vi "Handle Request.vi"(7 "Processing In":refnum<class "Processing.lvclass">, 11 "SSE Handler in":refnum<class "SSE Handler.lvclass">) -> (0 "error out":errorcluster, 5 "Processing":refnum<class "Processing.lvclass">)   [LabVIEW 2020, in "HTTP Server.lvlib" / "SSE Handler.lvclass"]
uses:
  SSE Handler.lvclass
  Processing/Processing.lvclass
  Processing/Processing.lvclass/Processing.ctl
  SSE Manager/SSE Manager.lvclass
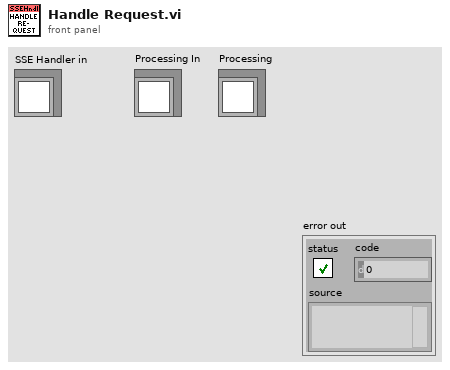
[diagram p1: front panel]
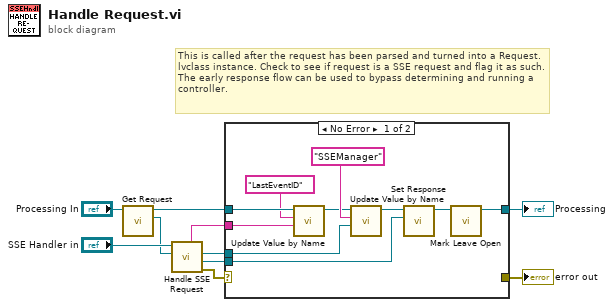
[diagram p0: block diagram]
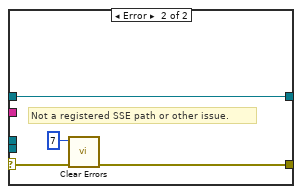
[diagram p2: hidden frame]
diagram:
  # "This is called after the request has been parsed and turned into a Request.lvclass instance. Check to see if request is a SSE request and flag it as such. The early response flow can be used to bypass determining and running a controller."
  n1 = call "Get Request.vi"("Processing in"="Processing In") -> ("Request"=w6:refnum<class "Request.lvclass">, "Processing out"=w9:refnum<class "Processing.lvclass">)  [unwired: 9 in]
  n2 = call "Handle SSE Request.vi"("Request"=w6, "SSE Handler in"="SSE Handler in") -> ("error out"=w5:errorcluster, "Response"=w4:refnum<class "Response.lvclass">, "SSE Manager"=w3:refnum<class "SSE Manager.lvclass">, "Last Event ID"=w2:string)  [unwired: 5 in, 1 out]
  n3 = case shown="No Error" w5 {
    selector: w5 -> [_ w23]
    tunnel: w4 -> [w17 _]
    tunnel: w9 -> [w14 w24]
    tunnel: [w16 w24] -> w8
    tunnel: w3 -> [w15 _]
    tunnel: w2 -> [w11 _]
    tunnel: [_ w21] -> w1
    frame No Error {
      n4 = call "Update Value by Name.vi"("Value"=w11, "Name"="LastEventID" ("Name / Service / Object"), "Processing in"=w14) -> ("Processing out"=w13:refnum<class "Processing.lvclass">)  [unwired: 7 in, 1 out]
      n5 = call "Update Value by Name.vi"("Value"=w15, "Name"="SSEManager" ("Name / Service / Object"), "Processing in"=w13) -> ("Processing out"=w19:refnum<class "Processing.lvclass">)  [unwired: 7 in, 1 out]
      n6 = call "Set Response.vi"("Response"=w17, "Processing in"=w19) -> ("Processing out"=w20:refnum<class "Processing.lvclass">)  [unwired: 9 in]
      n7 = call "Mark Leave Open.vi"("Processing in"=w20) -> ("Processing out"=w16:refnum<class "Processing.lvclass">)  [unwired: 10 in]
    }
    frame Error {
      # "Not a registered SSE path or other issue."
      n8 = call <vilib>:"Clear Errors.vi"("error in (no error)"=w23, "specific error code to clear (0: all)"=7) -> ("error out"=w21:errorcluster)  [unwired: 4 in, 1 out]
    }
  }
  "error out" <- w1
  "Processing" <- w8
